vi "LED_Command.vi"(4 "L lower limit":i32=25, 5 "Hue lower limit":i32=65, 6 "L upper limit":i32=70, 7 "Hue upper limit":i32=150, 8 "error in (no error)":errorcluster, 10 "channel":string, 11 "VISA resource in":refnum<visa-resource-name>) -> (0 "error out":errorcluster, 1 "read buffer":string, 2 "Result":bool, 3 "VISA resource out":refnum<visa-resource-name>)   [LabVIEW 2020]
uses:
  ac39a300-4e64-4893-9030-d78369e52789.vi
  <vilib>/Instr/_visa.llb/VISA Configure Serial Port (Instr).vi
panel:
  # "1 ,   2,  3,    4,   5,  6  ,7\nD3,D4,D5,D6,D7,D8,D9"
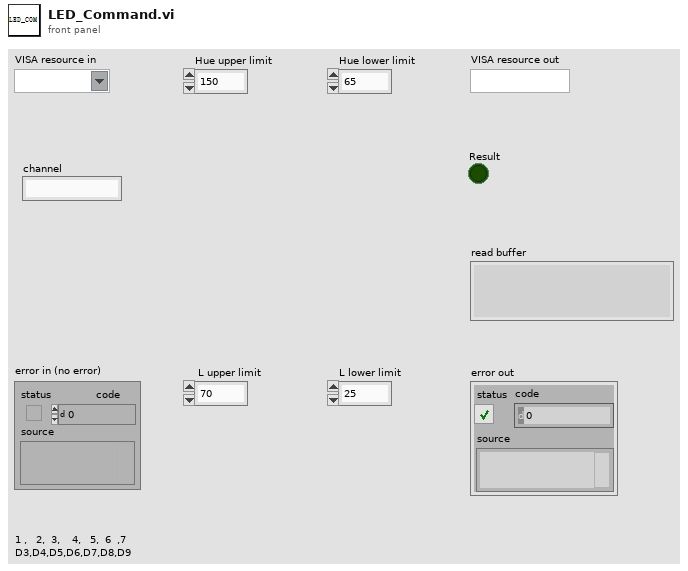
[diagram p1: front panel]
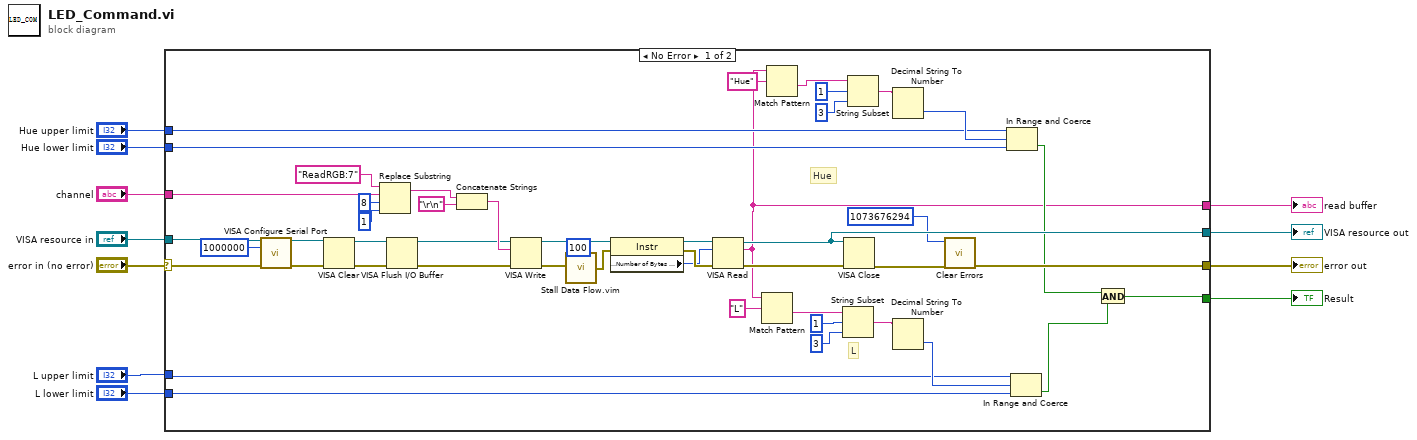
[diagram p0: block diagram]
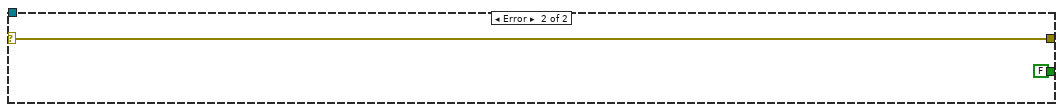
[diagram p2: hidden frame]
diagram:
  n1 = case shown="No Error" "error in (no error)" {
    selector: "error in (no error)" -> [w58 w61]
    tunnel: "VISA resource in" -> [w59 _]
    tunnel: [w56 _] -> w9
    tunnel: [w15 _] -> w8
    tunnel: [w30 w61] -> w7
    tunnel: "channel" -> [w36 _]
    tunnel: "L upper limit" -> [w23 _]
    tunnel: "L lower limit" -> [w22 _]
    tunnel: "Hue upper limit" -> [w21 _]
    tunnel: "Hue lower limit" -> [w20 _]
    tunnel: [w19 FALSE ("Result")] -> w1
    frame No Error {
      # "L"
      # "Hue"
      n2 = call-poly "VISA Configure Serial Port"("VISA resource name"=w59, "baud rate (9600)"=u32 1000000, "error in (no error)"=w58) -> ("VISA resource name out"=w43:refnum<visa-resource-name>, "error out"=w42:errorcluster)  [unwired: 11 in]
      n3 = VISA Clear(VISA resource name=w43, error in (no error)=w42) -> (VISA resource name out=w41:refnum<visa-resource-name>, error out=w40:errorcluster)
      n4 = Replace Substring(2:1 ("length (len. of substring)"), 3:8 ("offset (0)"), 4:w36, 5:"ReadRGB:7" ("write buffer")) -> (1:w33:string)  [unwired: 1 out]
      n5 = VISA Flush I/O Buffer(VISA resource name=w41, error in (no error)=w40) -> (VISA resource name out=w39:refnum<visa-resource-name>, error out=w38:errorcluster)  [unwired: 1 in]
      n6 = Concatenate Strings(w33, "\r\n") -> (w47:string)
      n7 = VISA Write(VISA resource name=w39, write buffer=w47, error in (no error)=w38) -> (VISA resource name out=w52:refnum<visa-resource-name>, error out=w46:errorcluster)  [unwired: 1 out]
      n8 = call "Stall Data Flow.vim"("value in"=w46, "milliseconds to wait"=u32 100) -> ("value out"=w45:errorcluster)  [unwired: 1 out]
      n9 = property class="Instr"(reference=w52, error in=w45) -> (reference out=w51:refnum<visa-resource-name>, error out=w50:errorcluster, "Serial Settings:Number of Bytes at Serial Port"=w49:u32)
      n10 = VISA Read(VISA resource name=w51, byte count=w49, error in (no error)=w50) -> (VISA resource name out=w56:refnum<visa-resource-name>, read buffer=w15:string, error out=w57:errorcluster)  [unwired: 1 out]
      n11 = Match Pattern(string=w15, regular expression="L") -> (after substring=w13:string)  [unwired: 1 in, 3 out]
      n12 = Match Pattern(string=w15, regular expression="Hue") -> (after substring=w12:string)  [unwired: 1 in, 3 out]
      n13 = String Subset(string=w13, offset (0)=1, length (rest)=3 ("length (rest)")) -> (substring=w28:string)
      n14 = VISA Close(VISA resource name=w56, error in (no error)=w57) -> (error out=w54:errorcluster)
      n15 = String Subset(string=w12, offset (0)=1, length (rest)=3 ("length (rest)")) -> (substring=w29:string)
      n16 = Decimal String To Number(string=w29) -> (number=w24:i32)  [unwired: 2 in, 1 out]
      n17 = Decimal String To Number(string=w28) -> (number=w25:i32)  [unwired: 2 in, 1 out]
      n18 = call <vilib>:"Clear Errors.vi"("error in (no error)"=w54, "specific error code to clear (0: all)"=1073676294) -> ("error out"=w30:errorcluster)  [unwired: 4 in, 1 out]
      n19 = In Range and Coerce(upper limit=w21, x=w24, lower limit=w20) -> (In Range?=w18:bool)  [unwired: 1 out]
      n20 = In Range and Coerce(upper limit=w23, x=w25, lower limit=w22) -> (In Range?=w17:bool)  [unwired: 1 out]
      n21 = And(x=w18, y=w17) -> (x .and. y?=w19:bool)
    }
    frame Error {
    }
  }
  "VISA resource out" <- w9
  "error out" <- w7
  "read buffer" <- w8
  "Result" <- w1
